vi "Day 3.2 - Gear Ratio.vi"(11 "input":string[](array[string])) -> (3 "ouptut part 2":u64)   [LabVIEW 2021]
uses:
  <vilib>/regexp/Match Regular Expression.xnode
panel:
  out "Array":string[](array[string])
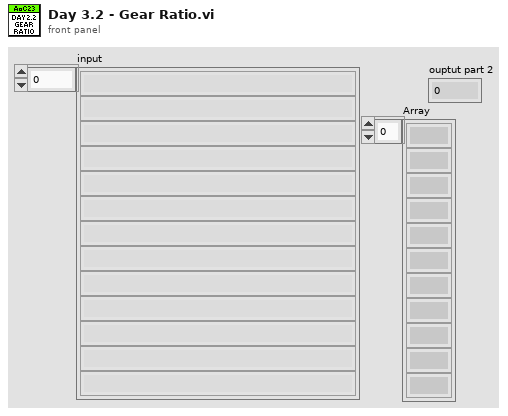
[diagram p1: front panel]
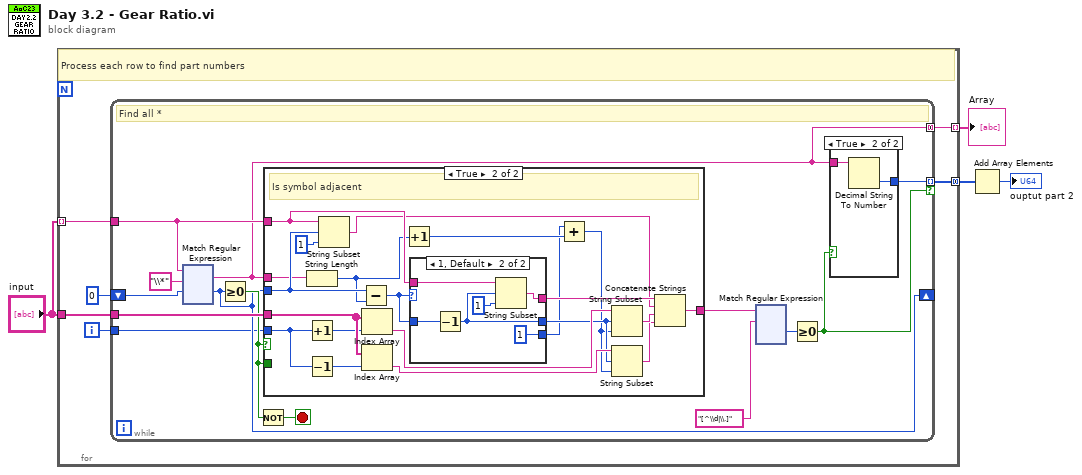
[diagram p0: block diagram]
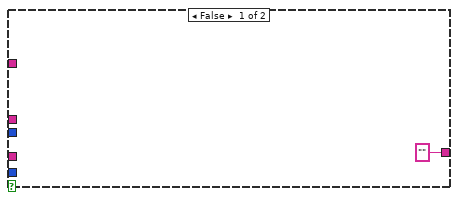
[diagram p3: hidden frame]
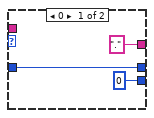
[diagram p4: hidden frame]
diagram:
  n1 = for {
    tunnel: "input" -> [w10] mode=indexing
    tunnel: "input" -> [w8]
    tunnel: [w6] -> w2 mode=concatenating
    tunnel: [w5] -> w1 mode=indexing
    i -> [w7]
    # "Process each row to find part numbers"
    n2 = while {
      tunnel: w10 -> [w20]
      tunnel: w8 -> [w21]
      shift-right: [w18] -> _
      shift-left: 0 -> [w22]
      tunnel: w7 -> [w17]
      tunnel: [w13] -> w6 mode=indexing if=w12
      tunnel: [w11] -> w5 mode=concatenating
      stop <- w23 stop-if-true
      # "Find all *"
      n3 = xnode "Match Regular Expression"("input string"=w20, "regular expression"="\\*", "offset (0)"=w22) -> ("whole match"=w11:string, "offset past match"=w18:i32)  [unwired: 3 in, 3 out]
      n4 = Greater Or Equal To 0?(x=w18) -> (x >= 0?=w19:bool)
      n5 = Not(x=w19) -> (.not. x?=w23:bool)
      n6 = case shown="True" w19 {
        tunnel: w11 -> [_ w158]
        tunnel: w19 -> [_ _]
        tunnel: w21 -> [_ w157]
        tunnel: w20 -> [_ w163]
        tunnel: ["" w165] -> w16
        tunnel: w18 -> [_ w160]
        tunnel: w17 -> [_ w154]
        frame False {
        }
        frame True {
          # "Is symbol adjacent"
          n7 = String Length(string=w158) -> (length=w147:i32)
          n8 = Increment(x=w154) -> (x+1=w156:i32)
          n9 = Decrement(x=w154) -> (x-1=w155:i32)
          n10 = String Subset(string=w163, offset (0)=w160, length (rest)=1 ("length (rest)")) -> (substring=w161:string)
          n11 = Subtract(x=w160, y=w147) -> (x-y=w159:i32)
          n12 = Index Array(array=w157, index=w156) -> (element=w153:string)
          n13 = Index Array(array=w157, index=w155) -> (element=w152:string)
          n14 = Increment(x=w147) -> (x+1=w151:i32)
          n15 = case shown="1, Default" w159 {
            tunnel: w163 -> [_ w174]
            tunnel: w159 -> [w167 w173]
            tunnel: ["." w171] -> w162
            tunnel: [w167 w170] -> w148
            tunnel: [0 1] -> w145
            frame 0 {
            }
            frame 1, Default {
              n16 = Decrement(x=w173) -> (x-1=w170:i32)
              n17 = String Subset(string=w174, offset (0)=w170, length (rest)=1 ("length (rest)")) -> (substring=w171:string)
            }
          }
          n18 = Add(x=w145, y=w151) -> (x+y=w146:i32)
          n19 = String Subset(string=w153, offset (0)=w148, length (rest)=w146) -> (substring=w150:string)
          n20 = String Subset(string=w152, offset (0)=w148, length (rest)=w146) -> (substring=w149:string)
          n21 = Concatenate Strings(w162, w161, w150, w149) -> (w165:string)
        }
      }
      n22 = xnode "Match Regular Expression"("input string"=w16, "regular expression"="[^\\d|\\.]") -> ("offset past match"=w14:i32)  [unwired: 4 in, 4 out]
      n23 = Greater Or Equal To 0?(x=w14) -> (x >= 0?=w12:bool)
      n24 = case shown="True" w12 {
        tunnel: w11 -> [_ w26]
        tunnel: [_ w25] -> w13
        frame False {
        }
        frame True {
          n25 = Decimal String To Number(string=w26) -> (number=w25:i32)  [unwired: 2 in, 1 out]
        }
      }
    }
  }
  "Array" <- w1
  n26 = Add Array Elements(numeric array=w2) -> (sum=→"ouptut part 2":i32)
